vi "_PC_Pub_Splitter_ResizeWindow.vi"(1 "sys_value_list":refnum<vi>, 2 "d999_list":refnum<vi>, 3 "Config Tab":refnum<vi>) -> ()   [LabVIEW 2018]
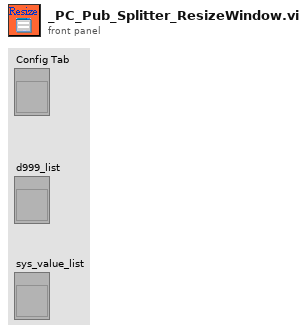
[diagram p1: front panel]
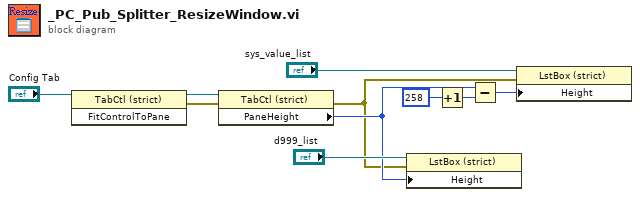
[diagram p0: block diagram]
diagram:
  n1 = invoke class="TabCtl (strict)" method="FitControlToPane"(reference="Config Tab") -> (reference out=w9:refnum<vi>, error out=w10:errorcluster)  [unwired: 2 in, 1 out]
  n2 = property class="TabCtl (strict)"(reference=w9, error in=w10) -> (error out=w1:errorcluster, "PaneHeight"=w3:u32)  [unwired: 1 out]
  n3 = property class="LstBox (strict)"(reference="d999_list", error in=w1, "Height"=w3) -> ()  [unwired: 2 out]
  n4 = Increment(x=u32 258 ("Height")) -> (x+1=w4:u32)
  n5 = Subtract(x=w3, y=w4) -> (x-y=w5:u32)
  n6 = property class="LstBox (strict)"(reference="sys_value_list", error in=w1, "Height"=w5) -> ()  [unwired: 2 out]
